vi "Try Match Response.vi"(8 "error in":errorcluster, 10 "ICAN CC Frame":refnum<class "ICAN CC Frame.lvclass">, 11 "Upload Transfer in":refnum<class "Upload Transfer.lvclass">) -> (0 "error out":errorcluster, 2 "Success":bool, 3 "SDO Transfer out":refnum<class "SDO Transfer.lvclass">)   [LabVIEW 2020, in "SDO Manager.lvlib" / "Upload Transfer.lvclass"]
uses:
  Upload Transfer.lvclass
  SDO Transfer/SDO Transfer.lvclass
  HAL/Source/Interfaces/ICAN CC Frame/ICAN CC Frame.lvclass
  Segmented Upload Transfer/Segmented Upload Transfer.lvclass
  HAL/Source/Interfaces/ICommunicate/ICommunicate.lvclass
  Upload Transfer.lvclass/Upload Transfer.ctl
  Typedefs/SDO Result.ctl
  CANopen.lvlib
  SDO Transfer/SDO abort code.ctl
  CANopen Message/CANopen Message.lvclass
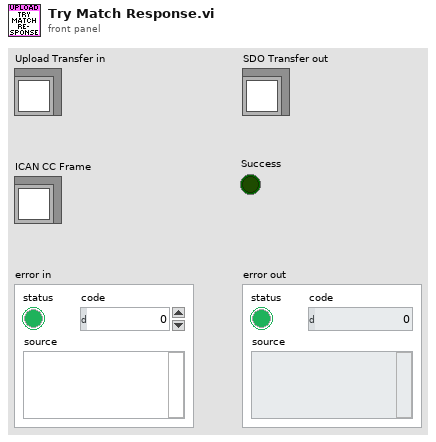
[diagram p1: front panel]
types:
  T1 = typedef "CANopen.lvlib/SDO Result.ctl" = cluster{"Success":bool, "SDO abort code":cluster{"Null":bool, "Value":T2}, "Data":cluster{"Null":bool, "Data":u8[]}}
  T2 = typedef "SDO Manager.lvlib/SDO Transfer.lvclass/SDO abort code.ctl" = u32
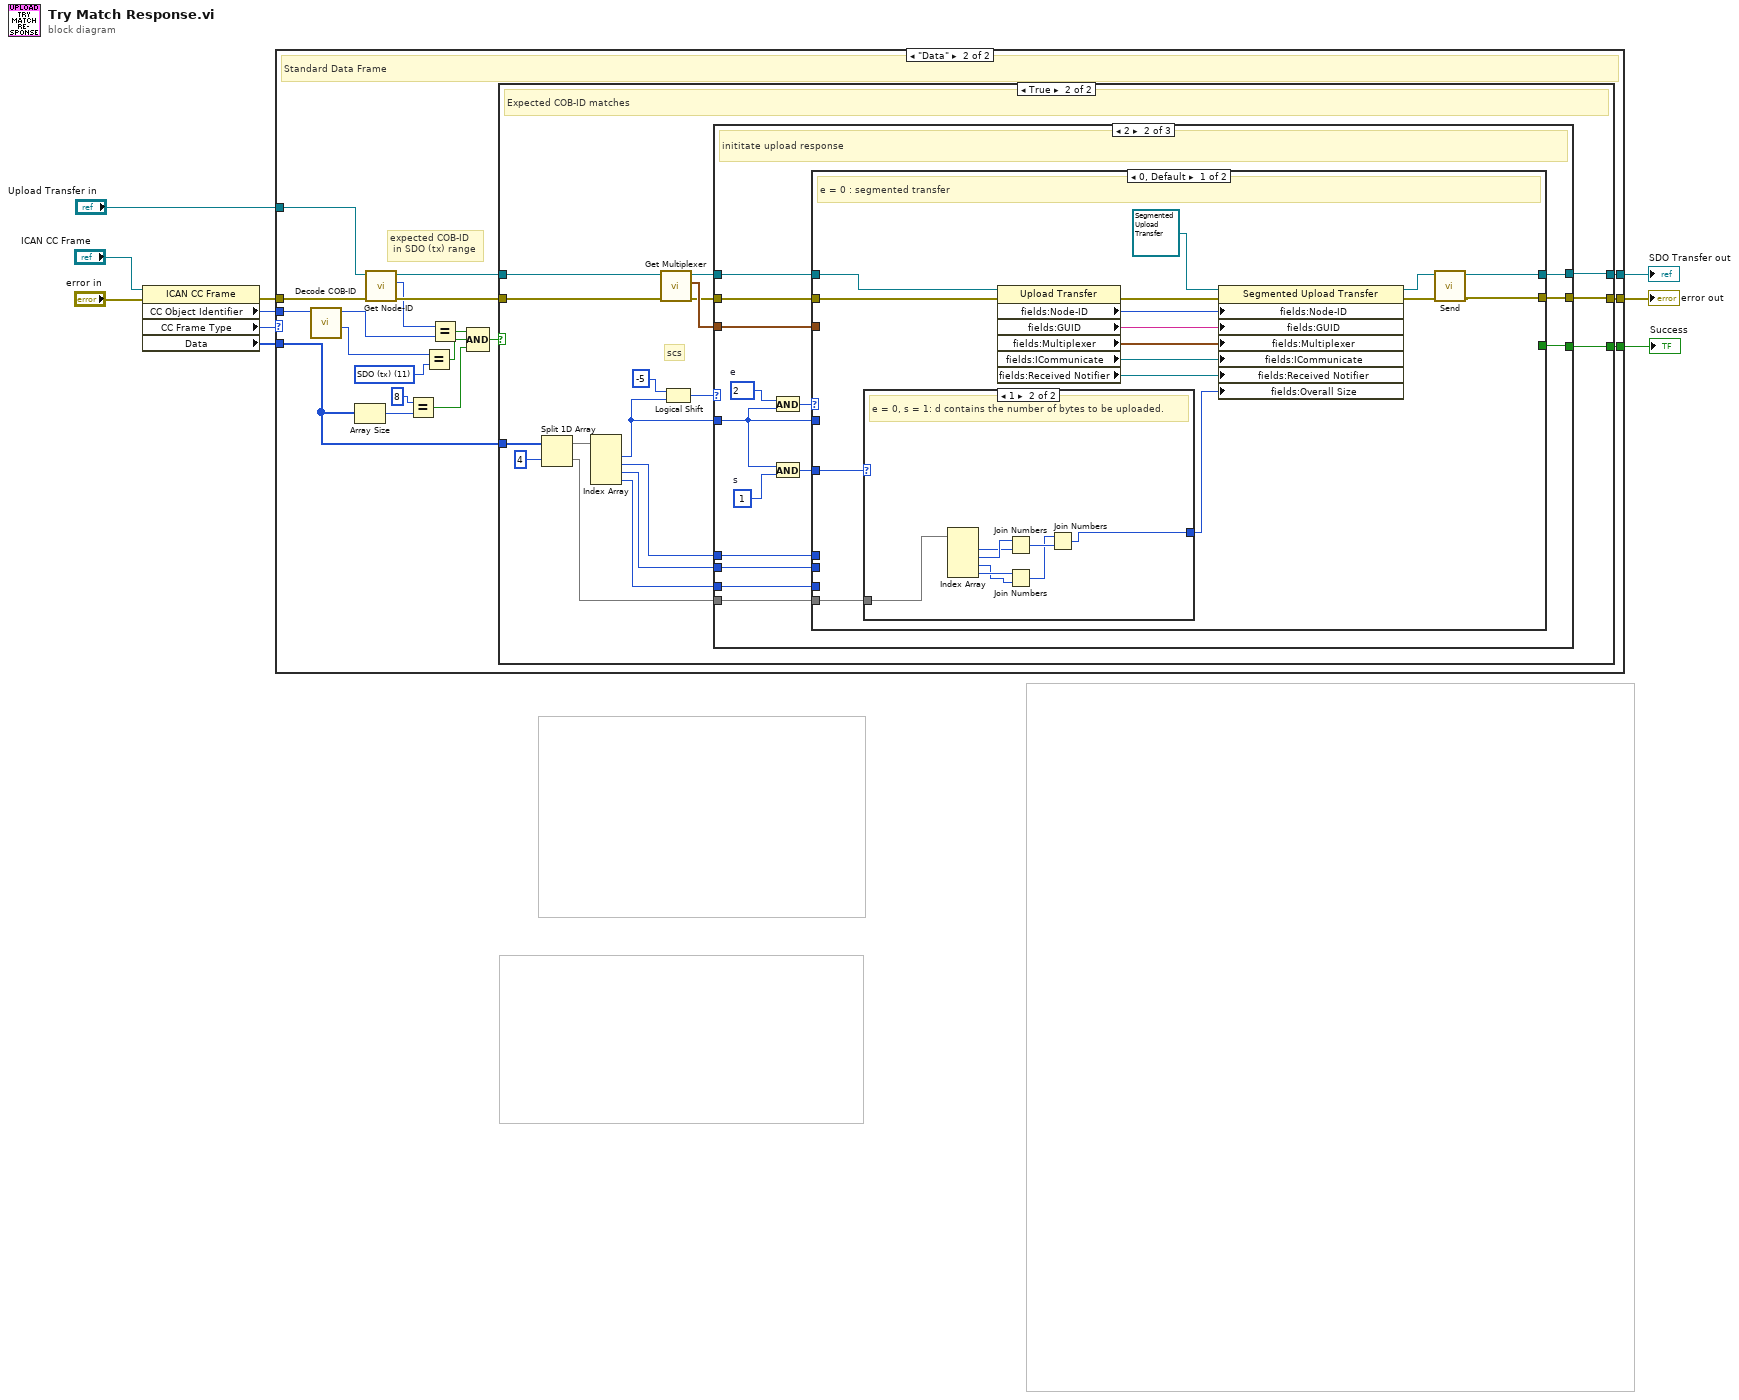
[diagram p0: block diagram]
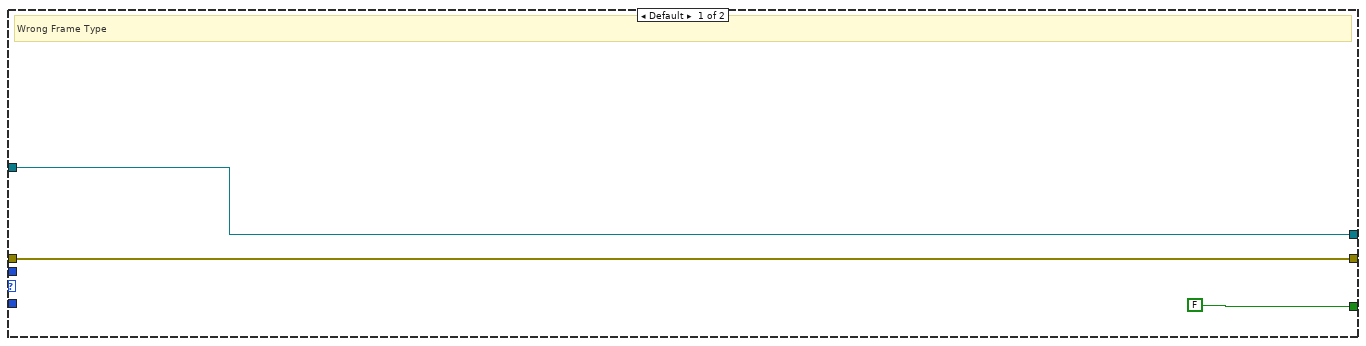
[diagram p2: hidden frame]
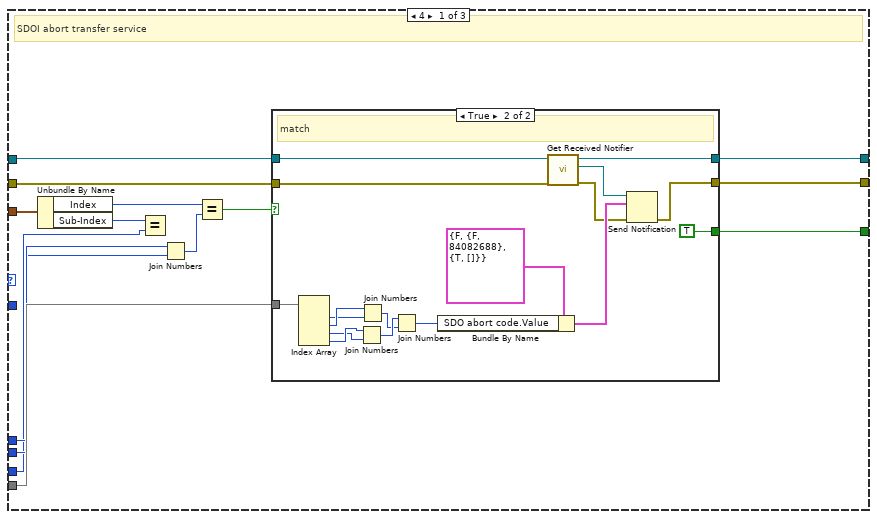
[diagram p4: hidden frame]
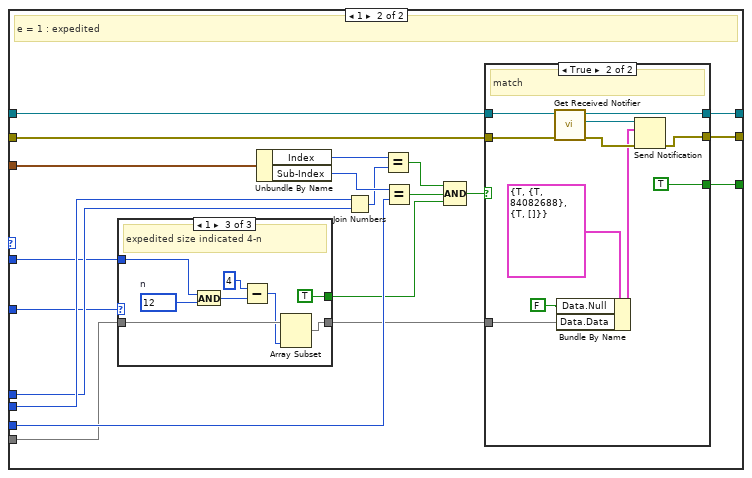
[diagram p7: hidden frame]
diagram:
  n1 = property class="ICAN CC Frame"(reference="ICAN CC Frame", error in="error in") -> (error out=w8:errorcluster, "CC Object Identifier"=w3:u32, "CC Frame Type"=w1:enum8{"Data", "Remote", "Error", "Overload"}, "Data"=w2:u8[])  [unwired: 1 out]
  n2 = case shown="\"Data\"" w1 {
    tunnel: w8 -> [w12 w32]
    tunnel: "Upload Transfer in" -> [w11 w31]
    tunnel: [w11 w28] -> w6
    tunnel: [w12 w27] -> w5
    tunnel: [FALSE w26] -> w4
    tunnel: w3 -> [_ w25]
    tunnel: w2 -> [_ w14]
    frame Default {
      # "Wrong Frame Type"
    }
    frame "Data" {
      w22 = u8 11 items=["NMT"=0, "EMCY/SYNC"=1, "TIME"=2, "PDO1 (tx)"=3, "PDO1 (rx)"=4, "PDO2 (tx)"=5, "PDO2 (rx)"=6, "PDO3 (tx)"=7, "PDO3 (rx)"=8, "PDO4 (tx)"=9, "PDO4 (rx)"=10, "SDO (tx)"=11, "SDO (rx)"=12, "NMT error control"=14] ("Function Code")
      # "expected COB-ID\n in SDO (tx) range"
      # "Standard Data Frame"
      n3 = call "Decode COB-ID.vi"("COD-ID"=w25) -> ("Function Code"=w21:u8, "Node-ID"=w24:u8)  [unwired: 9 in]
      n4 = Array Size(array=w14) -> (size(s)=w20:i32)
      n5 = call "Get Node-ID.vi"("error in"=w32, "SDO Transfer in"=w31) -> ("error out"=w29:errorcluster, "Node-ID"=w23:u8, "SDO Transfer out"=w30:refnum<class "Upload Transfer.lvclass">)  [unwired: 7 in]
      n6 = Equal?(x=8, y=w20) -> (x = y?=w15:bool)
      n7 = Equal?(x=w21, y=w22) -> (x = y?=w16:bool)
      n8 = Equal?(x=w23, y=w24) -> (x = y?=w17:bool)
      n9 = Compound Arithmetic op=AND(w17, w16, w15) -> (w18:bool)
      n10 = case shown="True" w18 {
        tunnel: w30 -> [w34 w51]
        tunnel: w29 -> [w33 w50]
        tunnel: [w34 w40] -> w28
        tunnel: [w33 w41] -> w27
        tunnel: w14 -> [_ w47]
        tunnel: [_ w39] -> w26
        frame False {
        }
        frame True {
          # "scs"
          # "Expected COB-ID matches"
          n11 = Split 1D Array(array=w47, index=4) -> (first subarray=w35:u8[], second subarray=w36:u8[])
          n12 = Index Array(array=w35) -> (element #1=w38:u8, element #2=w46:u8, element #3=w45:u8, element #4=w44:u8)  [unwired: 4 in]
          n13 = call "Get Multiplexer.vi"("error in"=w50, "SDO Transfer in"=w51) -> ("error out"=w42:errorcluster, "Multiplexer"=w48:cluster{"Index":u16, "Sub-Index":u8}, "SDO Transfer out"=w43:refnum<class "Upload Transfer.lvclass">)  [unwired: 7 in]
          n14 = Logical Shift(y=i16 -5, x=w38) -> (x << y=w49:u8)
          n15 = case shown="2" w49 {
            tunnel: w48 -> [w59 w100 _]
            tunnel: w46 -> [w57 w98 _]
            tunnel: w45 -> [w58 w99 _]
            tunnel: w44 -> [w55 w97 _]
            tunnel: w43 -> [w65 w94 w169]
            tunnel: w42 -> [w66 w96 w170]
            tunnel: [w64 w93 w169] -> w40
            tunnel: [w63 w95 w170] -> w41
            tunnel: [w62 w92 _] -> w39
            tunnel: w38 -> [_ w89 _]
            tunnel: w36 -> [w61 w91 _]
            frame 4 {
              # "SDOI abort transfer service"
              n16 = Unbundle By Name(w59) -> ("Index"=w60:u16, "Sub-Index"=w56:u8)
              n17 = Equal?(x=w56, y=w55) -> ()  [unwired: 1 out]
              n18 = Join Numbers(hi=w58, lo=w57) -> ((hi.lo)=w54:u16)
              n19 = Equal?(x=w60, y=w54) -> (x = y?=w53:bool)
              n20 = case shown="True" w53 {
                tunnel: w66 -> [w68 w83]
                tunnel: w65 -> [w67 w82]
                tunnel: [w67 w80] -> w64
                tunnel: [w68 w75] -> w63
                tunnel: [_ TRUE] -> w62
                tunnel: w61 -> [_ w73]
                frame False {
                  # "no match"
                }
                frame True {
                  # "match"
                  n21 = Index Array(array=w73) -> (element #1=w69:u8, element #2=w70:u8, element #3=w71:u8, element #4=w72:u8)  [unwired: 4 in]
                  n22 = Join Numbers(hi=w72, lo=w71) -> ((hi.lo)=w85:u16)
                  n23 = Join Numbers(hi=w70, lo=w69) -> ((hi.lo)=w84:u16)
                  n24 = Join Numbers(hi=w85, lo=w84) -> ((hi.lo)=w78:u32)
                  n25 = Bundle By Name(cluster=T1 {"Success"=FALSE, "SDO abort code"={"Null"=FALSE, "Value"=84082688}, "Data"={"Null"=TRUE, "Data"=[]}} ("notification"), "SDO abort code.Value"=w78) -> (w79:T1)
                  n26 = call "Get Received Notifier.vi"("error in"=w83, "SDO Transfer in"=w82) -> ("error out"=w76:errorcluster, "Received Notifier"=w81:refnum<notifier>, "SDO Transfer out"=w80:refnum<class "Upload Transfer.lvclass">)  [unwired: 7 in]
                  n27 = Send Notification(notification=w79, notifier=w81, error in (no error)=w76) -> (error out=w75:errorcluster)  [unwired: 1 out]
                }
              }
            }
            frame 2 {
              w87 = u8 1  # s
              w90 = u8 2  # e
              # "inititate upload response"
              n28 = And(x=w90, y=w89) -> (x .and. y?=w88:u8)
              n29 = And(x=w89, y=w87) -> (x .and. y?=w86:u8)
              n30 = case shown="0, Default" w88 {
                tunnel: w100 -> [_ w141]
                tunnel: w99 -> [_ w138]
                tunnel: w98 -> [_ w137]
                tunnel: w97 -> [_ w136]
                tunnel: w96 -> [w111 w135]
                tunnel: [w108 w134] -> w95
                tunnel: w94 -> [w116 w133]
                tunnel: [w107 w132] -> w93
                tunnel: w89 -> [_ w125]
                tunnel: [_ w128] -> w92
                tunnel: w91 -> [w114 w127]
                tunnel: w86 -> [w115 w126]
                frame 0, Default {
                  # "e = 0 : segmented transfer"
                  n31 = case shown="1" w115 {
                    tunnel: w114 -> [_ w124]
                    tunnel: [_ w117] -> w102
                    frame 0, Default {
                    }
                    frame 1 {
                      # "e = 0, s = 1: d contains the number of bytes to be uploaded."
                      n32 = Index Array(array=w124) -> (element #1=w120:u8, element #2=w121:u8, element #3=w122:u8, element #4=w123:u8)  [unwired: 4 in]
                      n33 = Join Numbers(hi=w121, lo=w120) -> ((hi.lo)=w119:u16)
                      n34 = Join Numbers(hi=w123, lo=w122) -> ((hi.lo)=w118:u16)
                      n35 = Join Numbers(hi=w118, lo=w119) -> ((hi.lo)=w117:u32)
                    }
                  }
                  n36 = property class="Upload Transfer"(reference=w116, error in=w111) -> (error out=w112:errorcluster, "fields:Node-ID"=w103:u8, "fields:GUID"=w101:string, "fields:Multiplexer"=w104:cluster{"Index":u16, "Sub-Index":u8}, "fields:ICommunicate"=w105:refnum<class "ICommunicate.lvclass">, "fields:Received Notifier"=w106:refnum<notifier>)  [unwired: 1 out]
                  n37 = property class="Segmented Upload Transfer"(reference=refnum<class "Segmented Upload Transfer.lvclass"> refnum ("CANopen Master:Segmented Upload Transfer.lvclass"), error in=w112, "fields:Node-ID"=w103, "fields:GUID"=w101, "fields:Multiplexer"=w104, "fields:ICommunicate"=w105, "fields:Received Notifier"=w106, "fields:Overall Size"=w102) -> (reference out=w109:refnum<class "Segmented Upload Transfer.lvclass">, error out=w110:errorcluster)
                  n38 = call-dynamic "Send.vi"("error in"=w110, "Segmented Upload Transfer"=w109) -> ("error out"=w108:errorcluster, "Segmented Upload Transfer"=w107:refnum<class "Segmented Upload Transfer.lvclass">)  [unwired: 8 in]
                }
                frame 1 {
                  # "e = 1 : expedited"
                  n39 = case shown="1" w126 {
                    tunnel: [w145 w146 w154] -> w130
                    tunnel: [_ TRUE TRUE] -> w129
                    tunnel: w127 -> [w145 w146 w155]
                    tunnel: w125 -> [_ _ w150]
                    frame Default {
                      # "not expedited"
                    }
                    frame 2 {
                      # "expedited, size not specified"
                    }
                    frame 1 {
                      w149 = u8 12  # n
                      # "expedited size indicated 4-n"
                      n40 = And(x=w150, y=w149) -> (x .and. y?=w148:u8)
                      n41 = Subtract(x=u8 4, y=w148) -> (x-y=w152:u8)
                      n42 = Array Subset(array=w155, length=w152) -> (w154:u8[])  [unwired: 1 in]
                    }
                  }
                  n43 = Unbundle By Name(w141) -> ("Index"=w142:u16, "Sub-Index"=w144:u8)
                  n44 = Join Numbers(hi=w138, lo=w137) -> ((hi.lo)=w143:u16)
                  n45 = Equal?(x=w142, y=w143) -> (x = y?=w140:bool)
                  n46 = Equal?(x=w144, y=w136) -> (x = y?=w139:bool)
                  n47 = Compound Arithmetic op=AND(w140, w139, w129) -> (w131:bool)
                  n48 = case shown="True" w131 {
                    tunnel: w135 -> [w157 w168]
                    tunnel: [w157 w167] -> w134
                    tunnel: w133 -> [w156 w164]
                    tunnel: [w156 w162] -> w132
                    tunnel: w130 -> [_ w158]
                    tunnel: [_ TRUE] -> w128
                    frame False {
                      # "no match"
                    }
                    frame True {
                      # "match"
                      n49 = call "Get Received Notifier.vi"("error in"=w168, "SDO Transfer in"=w164) -> ("error out"=w165:errorcluster, "Received Notifier"=w163:refnum<notifier>, "SDO Transfer out"=w162:refnum<class "Upload Transfer.lvclass">)  [unwired: 7 in]
                      n50 = Bundle By Name(cluster=T1 {"Success"=TRUE, "SDO abort code"={"Null"=TRUE, "Value"=84082688}, "Data"={"Null"=TRUE, "Data"=[]}} ("notification"), "Data.Null"=FALSE, "Data.Data"=w158) -> (w160:T1)
                      n51 = Send Notification(notification=w160, notifier=w163, error in (no error)=w165) -> (error out=w167:errorcluster)  [unwired: 1 out]
                    }
                  }
                }
              }
            }
            frame Default {
              # "scs no match"
            }
          }
        }
      }
    }
  }
  "SDO Transfer out" <- w6
  "error out" <- w5
  "Success" <- w4
